vi "level_probe_forhere.vi"(5 "Run VI":bool, 6 "Set # of Turns Open (Man)":dbl, 7 "Target Level (Auto)":dbl format="%.2f", 8 "stop":bool, 9 "Mode":enum32{"AUTOMATIC", "MANUAL"}(radio)=enum."MANUAL", 10 "position":refnum<vi>, 11 "level":refnum<vi>) -> ()   [LabVIEW 2015]
uses:
  <vilib>/Utility/config.llb/Read Key (String).vi
  <vilib>/Utility/config.llb/Read Key (Path).vi
  <vilib>/Utility/file.llb/Read Delimited Spreadsheet (DBL).vi
  <vilib>/Utility/file.llb/Write Delimited Spreadsheet (DBL).vi
  subvi_motor/global_motor.vi
  <vilib>/addons/control/pid/NI_PID_autopid.lvlib
  <vilib>/Utility/config.llb/NI_LVConfig.lvlib
panel:
  out "read buffer":string
  in  "Mode 2":enum32{"Continuous", "Sample and Hold"}(radio)
  in  "Motor Enabled":bool=TRUE
  out "levelbuffer":string
  out "Level":dbl(slide) scale=0.0..100.0
  in  "Save PID gains":bool
  in  "Load PID gains":bool
  in  "Recalibrate":bool
  in  "Current Position":dbl
  out "Motor Connected":bool
  in  "Enable Advanced Controls":bool
  in  "Log Data?":bool
  out "maxsteps":dbl
  out "minsteps":dbl
  in  "Min Open (Auto)":dbl=0.25
  in  "Max Open (Auto)":dbl=0.75
  out "Level":dynamicdata(graph)
  out "Error":dynamicdata(graph)
  in  "PID gains":T1={"proportional gain (Kc)"=10.0, "integral time (Ti, min)"=0.002, "derivative time (Td, min)"=0.2} {"derivative time (Td, min)" format="%.3f"; "integral time (Ti, min)" format="%.3f"; "proportional gain (Kc)" format="%.3f"}
  out "Valve Position":dynamicdata(graph)
  out "# of Turns Open":dbl
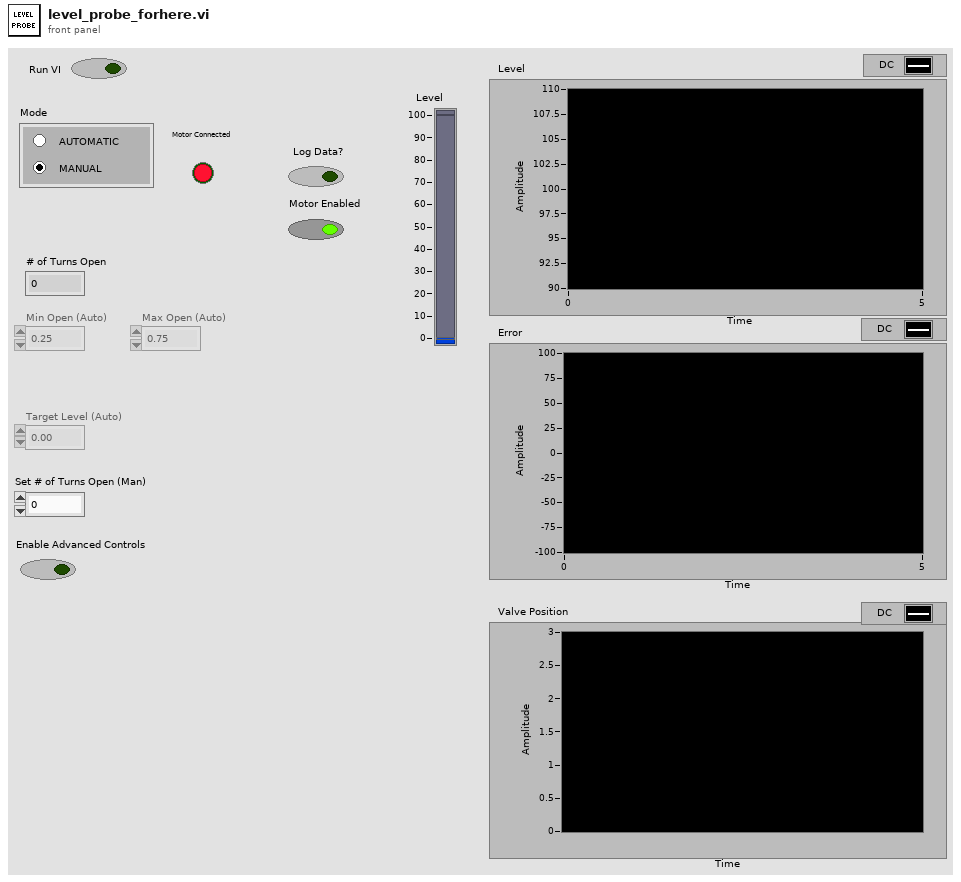
[diagram p1: front panel]
types:
  T1 = cluster{"proportional gain (Kc)":dbl, "integral time (Ti, min)":dbl, "derivative time (Td, min)":dbl}
  T2 = enum16{"open", "replace", "create", "open or create", "replace or create", "replace or create with confirmation"}
  T3 = enum8{"Enabled", "Disabled", "Disabled and Grayed Out"}
  T4 = typedef "NI_LVConfig.lvlib/Config Data RefNum.ctl" = refnum<k1>
  T5 = cluster{"first row[0]":dbl, "first row[1]":dbl, "first row[2]":dbl, "first row[3]":dbl, "first row[4]":dbl, "first row[5]":dbl, "first row[6]":dbl, "first row[7]":dbl, "first row[8]":dbl}
  T6 = cluster{"first row[0]":dbl, "first row[1]":dbl, "first row[2]":dbl}
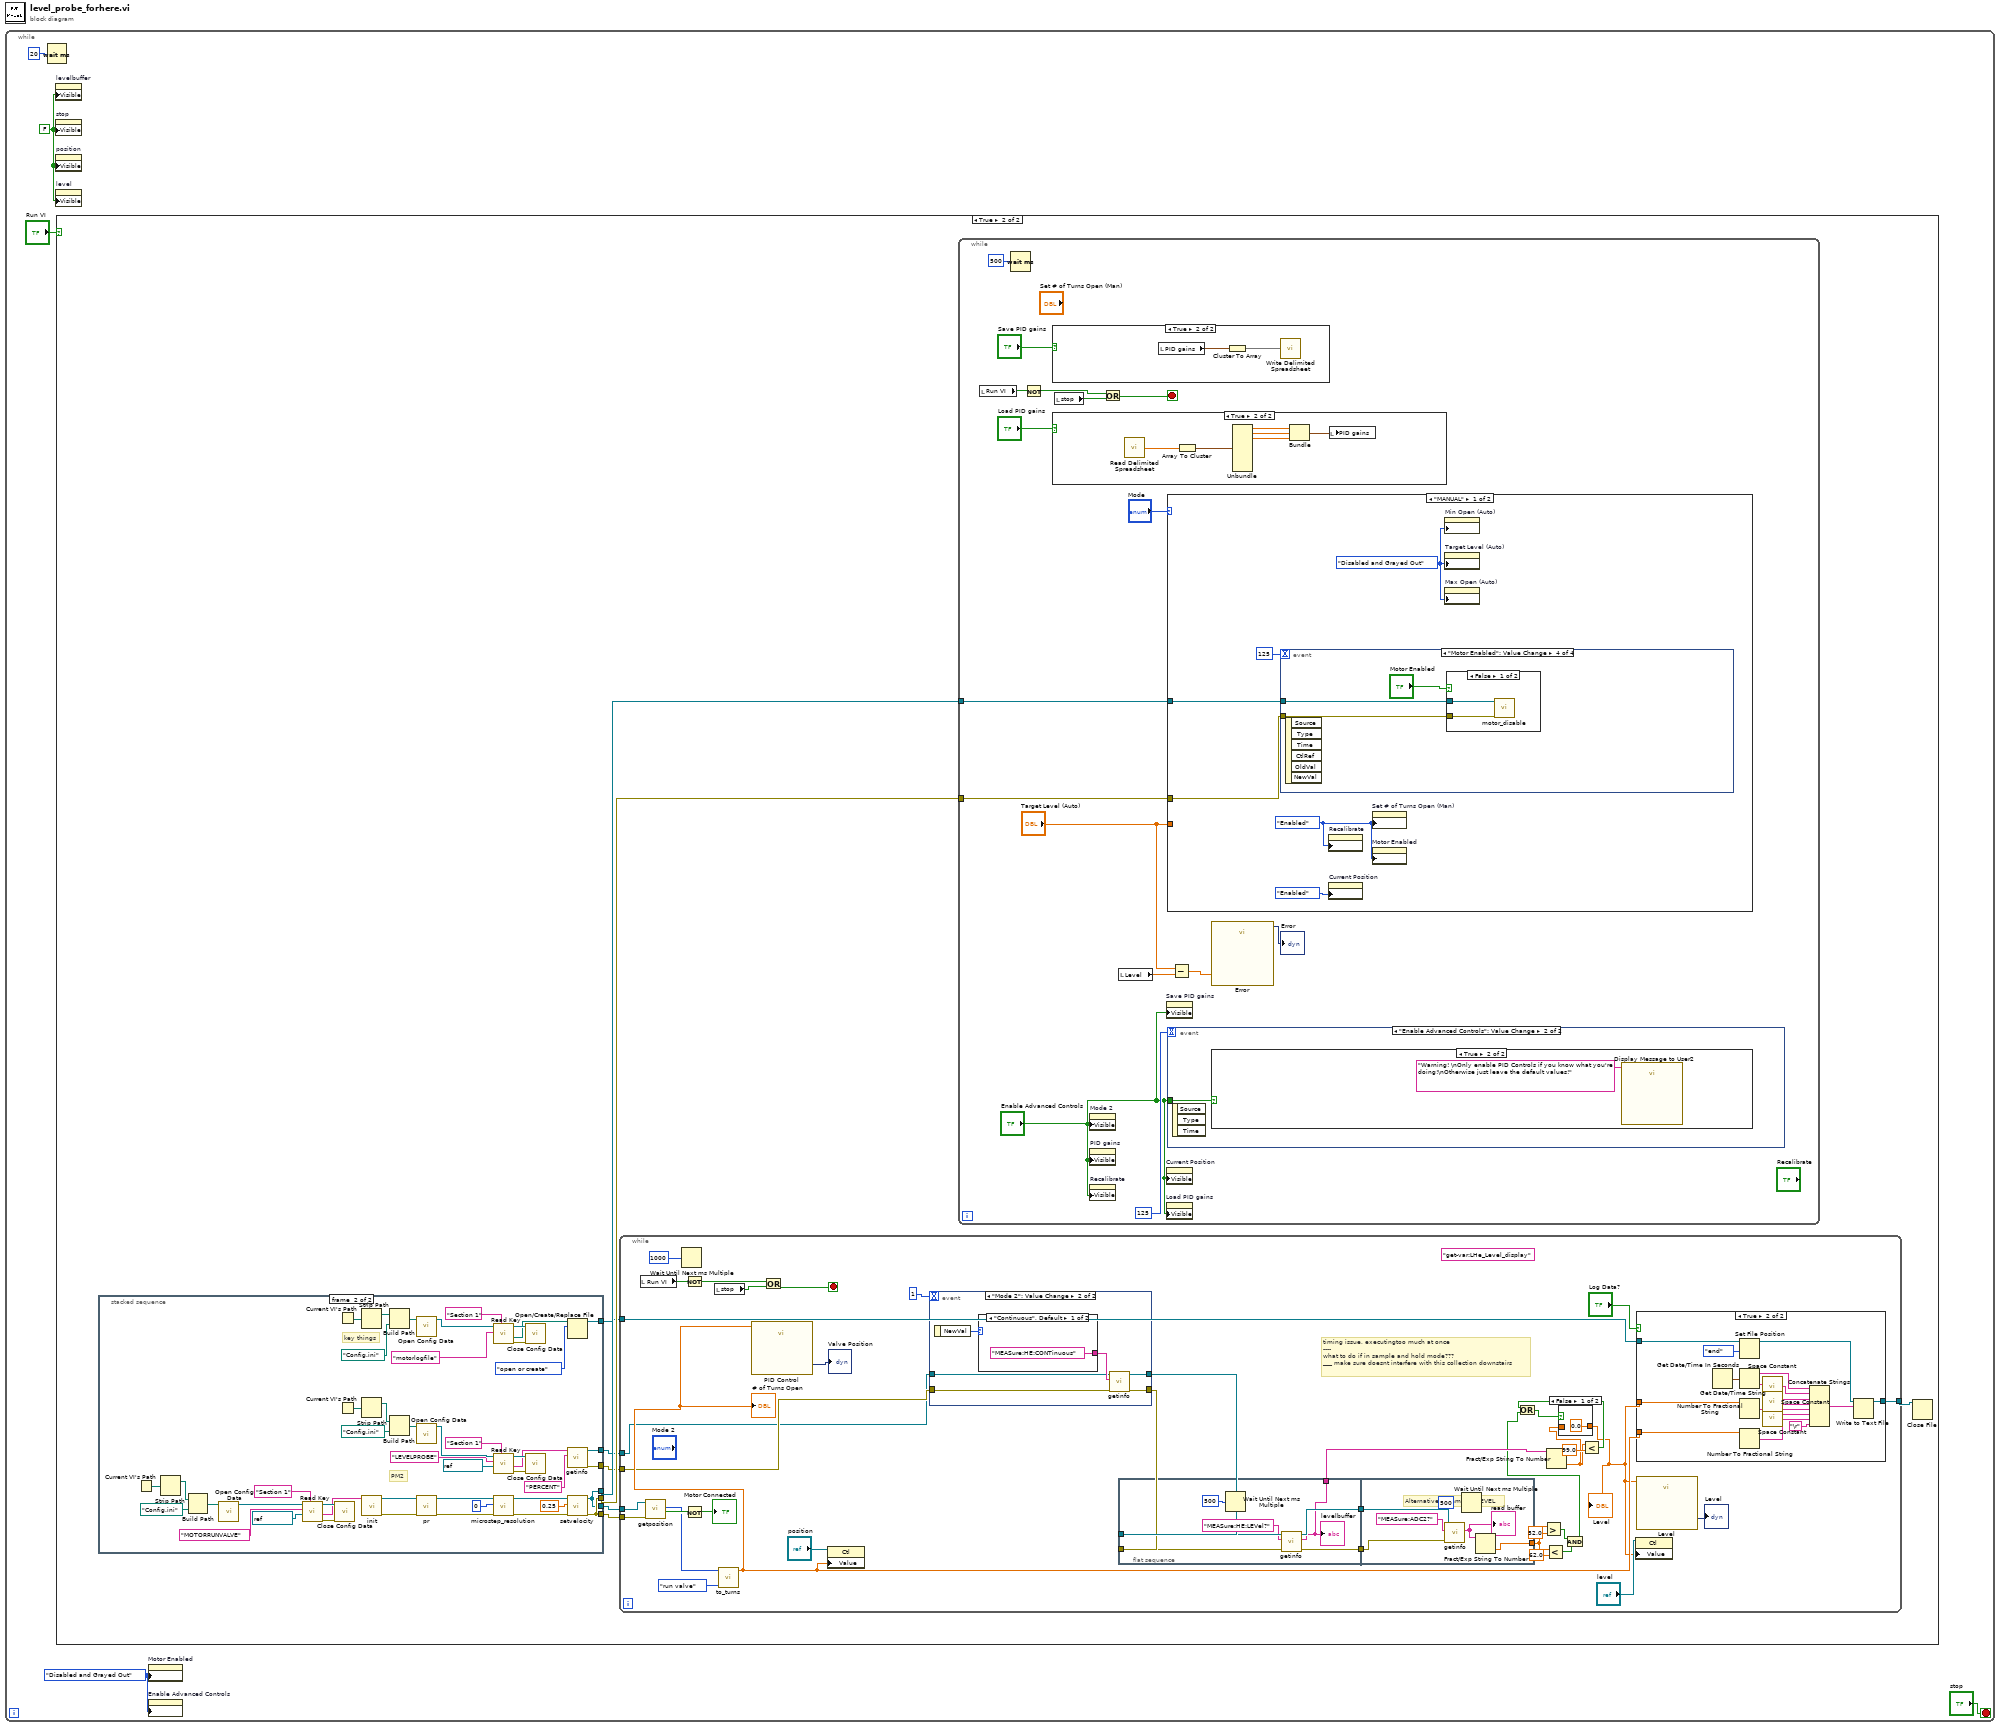
[diagram p0: block diagram]
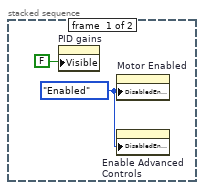
[diagram p3: hidden frame]
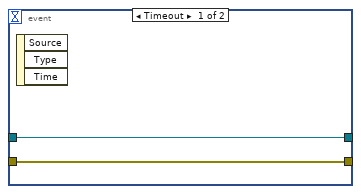
[diagram p5: hidden frame]
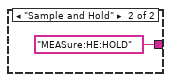
[diagram p6: hidden frame]
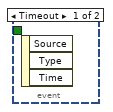
[diagram p8: hidden frame]
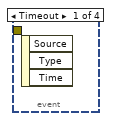
[diagram p12: hidden frame]
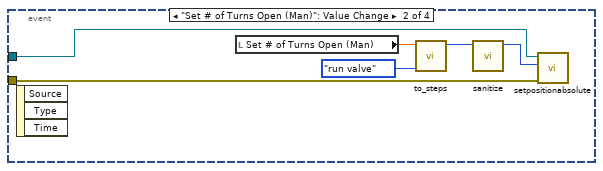
[diagram p13: hidden frame]
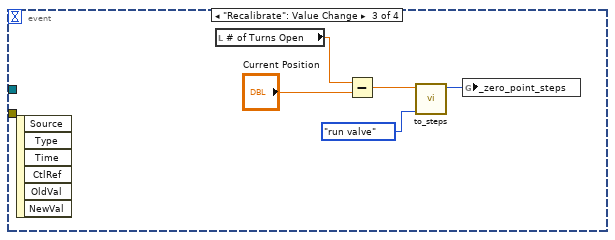
[diagram p14: hidden frame]
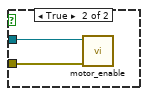
[diagram p15: hidden frame]
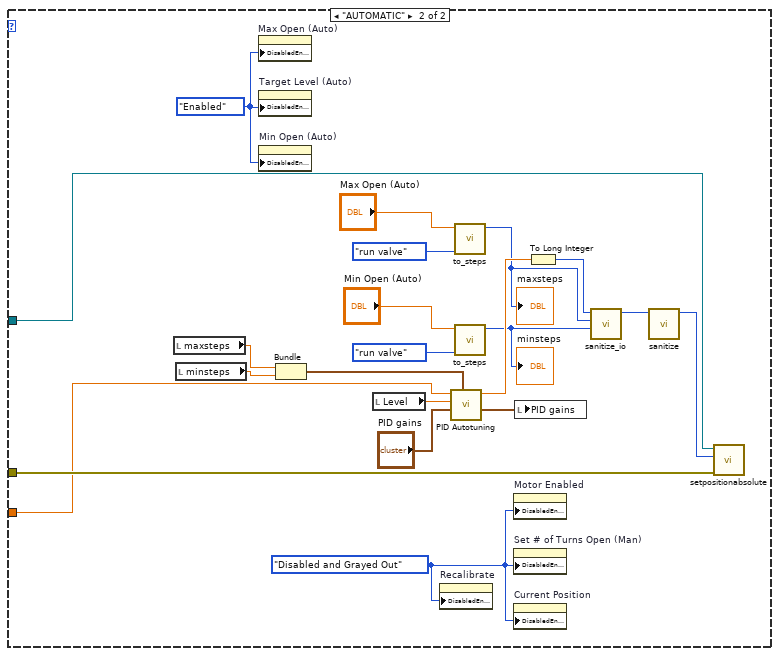
[diagram p16: hidden frame]
diagram:
  n1 = while {
    stop <- "stop" stop-if-true
    w1 = FALSE ("Visible")
    w2 = T3."Disabled and Grayed Out" ("Disabled")
    n2 = Wait (ms)(milliseconds to wait=u32 20) -> ()  [unwired: 1 out]
    n3 = property on="levelbuffer" class="Str"("Visible"=w1) -> ()  [unwired: 2 in, 2 out]
    n4 = property on="stop" class="Bool (strict)"("Visible"=w1) -> ()  [unwired: 2 in, 2 out]
    n5 = property on="position" class="LVObjRef (strict)"("Visible"=w1) -> ()  [unwired: 2 in, 2 out]
    n6 = property on="level" class="LVObjRef (strict)"("Visible"=w1) -> ()  [unwired: 2 in, 2 out]
    n7 = case shown="True" "Run VI" {
      frame False {
      }
      frame True {
        n8 = stacked-sequence {
          tunnel: [_ w61] -> w13
          tunnel: [_ w61] -> w12
          tunnel: [_ w60] -> w11
          tunnel: [_ w60] -> w10
          tunnel: [_ w55] -> w9
          tunnel: [_ w54] -> w8
          tunnel: [_ w53] -> w7
          frame #0 {
            w14 = T3."Enabled" ("Disabled")
            n9 = property on="PID gains" class="Clust (strict)"("Visible"=FALSE) -> ()  [unwired: 2 in, 2 out]
            n10 = property on="Motor Enabled" class="Bool (strict)"("DisabledEnum"=w14) -> ()  [unwired: 2 in, 2 out]
            n11 = property on="Enable Advanced Controls" class="Bool (strict)"("DisabledEnum"=w14) -> ()  [unwired: 2 in, 2 out]
          }
          frame #1 {
            # "PM2"
            # "key things"
            n12 = Current VI's Path() -> (path=w39:path)
            n13 = Strip Path(path=w39) -> (stripped path=w38:path)  [unwired: 1 out]
            n14 = Build Path(base path=w38, name or relative path=path "Config.ini" ("default name")) -> (appended path=w42:path)
            n15 = call <vilib>:"Open Config Data.vi"("configuration file path"=w42) -> ("refnum"=w47:T4)  [unwired: 8 in, 2 out]
            n16 = call-poly <vilib>:"Read Key.vi"("section"="Section 1", "default value"=refnum<visa-resource-name> "COM5" ("VISA resource name"), "key"="MOTORRUNVALVE", "refnum"=w47) -> ("error out"=w41:errorcluster, "value"=w37:string, "refnum out"=w45:T4)  [unwired: 4 in, 1 out]
            n17 = call <vilib>:"Close Config Data.vi"("error in (no error)"=w41, "refnum"=w45) -> ()  [unwired: 8 in, 2 out]
            n18 = Current VI's Path() -> (path=w19:path)
            n19 = Current VI's Path() -> (path=w28:path)
            n20 = Strip Path(path=w19) -> (stripped path=w18:path)  [unwired: 1 out]
            n21 = Strip Path(path=w28) -> (stripped path=w27:path)  [unwired: 1 out]
            n22 = call "init.vi"("VISA resource name"=w37) -> ("error out"=w49:errorcluster, "VISA resource name 2"=w51:refnum<visa-resource-name>)  [unwired: 9 in]
            n23 = Build Path(base path=w18, name or relative path=path "Config.ini" ("default name")) -> (appended path=w21:path)
            n24 = Build Path(base path=w27, name or relative path=path "Config.ini" ("default name")) -> (appended path=w31:path)
            n25 = call <vilib>:"Open Config Data.vi"("configuration file path"=w21) -> ("refnum"=w26:T4)  [unwired: 8 in, 2 out]
            n26 = call <vilib>:"Open Config Data.vi"("configuration file path"=w31) -> ("refnum"=w36:T4)  [unwired: 8 in, 2 out]
            n27 = call "pr.vi"("error in (no error)"=w49, "VISA resource name"=w51) -> ("error out"=w48:errorcluster, "VISA resource name 2"=w50:refnum<visa-resource-name>)  [unwired: 8 in]
            n28 = call-poly <vilib>:"Read Key.vi"("section"="Section 1", "key"="motorlogfile", "refnum"=w26) -> ("error out"=w20:errorcluster, "value"=w17:path, "refnum out"=w24:T4)  [unwired: 5 in, 1 out]
            n29 = call-poly <vilib>:"Read Key.vi"("section"="Section 1", "default value"=refnum<visa-resource-name> "COM8" ("VISA resource name"), "key"="LEVELPROBE", "refnum"=w36) -> ("error out"=w30:errorcluster, "value"=w16:string, "refnum out"=w34:T4)  [unwired: 4 in, 1 out]
            n30 = call "microstep_resolution.vi"("error in (no error)"=w48, "number"=0, "VISA in"=w50) -> ("error out"=w58:errorcluster, "VISA out"=w57:refnum<visa-resource-name>)  [unwired: 7 in]
            n31 = call <vilib>:"Close Config Data.vi"("error in (no error)"=w20, "refnum"=w24) -> ()  [unwired: 8 in, 2 out]
            n32 = call <vilib>:"Close Config Data.vi"("error in (no error)"=w30, "refnum"=w34) -> ()  [unwired: 8 in, 2 out]
            n33 = Open/Create/Replace File(file path (use dialog)=w17, operation (0:open)=T2."open or create") -> (refnum out=w53:refnum<file>)  [unwired: 4 in, 2 out]
            n34 = call "getinfo.vi"("string"="PERCENT", "VISA resource name"=w16) -> ("error out"=w54:errorcluster, "VISA resource name 2"=w55:refnum<visa-resource-name>)  [unwired: 7 in, 1 out]
            n35 = call "setvelocity.vi"("error in (no error)"=w58, "Velocity"=0.25, "VISA in"=w57) -> ("error out"=w61:errorcluster, "VISA out"=w60:refnum<visa-resource-name>)  [unwired: 7 in]
          }
        }
        n36 = while {
          tunnel: w12 -> [w100]
          tunnel: w10 -> [w99]
          tunnel: w9 -> [w80]
          tunnel: w8 -> [w81]
          tunnel: w7 -> [w85]
          tunnel: [w84] -> w6
          stop <- w87 stop-if-true
          (unwired) "get-var:LHe_Level_display" ("string")
          # "timing issue, executingtoo much at once\n----\nwhat to do if in sample and hold mode???\n___ make sure doesnt interfere with this collection downstairs"
          # "Alternative Command: LEVEL"
          n37 = local read "Run VI"() -> (w92:bool)
          n38 = call "getposition.vi"("error in (no error)"=w100, "VISA resource name"=w99) -> ("Is Null?"=w95:bool, "Position"=w93:i32)  [unwired: 6 in, 2 out]
          n39 = Wait Until Next ms Multiple(millisecond multiple=u32 1000 ("milliseconds to wait")) -> ()  [unwired: 1 out]
          n40 = Not(x=w92) -> (.not. x?=w88:bool)
          n41 = Not(x=w95) -> (.not. x?=→"Motor Connected":bool)
          n42 = local read "stop"() -> (w86:bool)
          n43 = call "to_turns.vi"("Radio Buttons"=enum32{"run valve", "bypass valve"}."run valve", "Steps"=w93) -> ("Turns"=w89:dbl)  [unwired: 9 in]
          "# of Turns Open" <- w89
          n44 = call "PID Control"("Offset"=w89) -> ("DC"=→"Valve Position":dynamicdata)  [unwired: 13 in, 1 out]
          n45 = Or(x=w88, y=w86) -> (x .or. y?=w87:bool)
          n46 = property class="Ctl"(reference="position", "Value"=w89) -> ()  [unwired: 1 in, 2 out]
          n47 = event shown="[1] \"Mode 2\": Value Change" {
            selector: _ -> [_ _]
            dyn-events: _ -> [_ _]
            timeout: 1 -> [_ _]
            tunnel: w81 -> [w116 w120]
            tunnel: w80 -> [w117 w121]
            tunnel: [w117 w119] -> w79
            tunnel: [w116 w118] -> w78
            event Timeout {
              n48 = event-data() -> ()  [unwired: 1 in, 3 out]
            }
            event "Mode 2": Value Change {
              n49 = event-data() -> ("NewVal"=w123:enum32{"Continuous", "Sample and Hold"})  [unwired: 1 in]
              n50 = case shown="\"Continuous\", Default" w123 {
                tunnel: ["MEASure:HE:CONTinuous" ("string") "MEASure:HE:HOLD"] -> w122
                frame "Continuous", Default {
                }
                frame "Sample and Hold" {
                }
              }
              n51 = call "getinfo.vi"("error in (no error)"=w120, "string"=w122, "VISA resource name"=w121) -> ("error out"=w118:errorcluster, "VISA resource name 2"=w119:refnum<visa-resource-name>)  [unwired: 6 in, 1 out]
            }
          }
          n52 = flat-sequence {
            tunnel: w79 -> [w109]
            tunnel: w78 -> [w107]
            tunnel: [w105] -> w76
            tunnel: [w104] -> w75
            tunnel: [w103] -> w74
            tunnel: w76 -> [w114]
            tunnel: w75 -> [w113]
            tunnel: [w110] -> w72
            frame #0 {
              n53 = Wait Until Next ms Multiple(millisecond multiple=u32 500) -> ()  [unwired: 1 out]
              n54 = call "getinfo.vi"("error in (no error)"=w107, "string"="MEASure:HE:LEVel?", "VISA resource name"=w109) -> ("error out"=w104:errorcluster, "read buffer"=w103:string, "VISA resource name 2"=w105:refnum<visa-resource-name>)  [unwired: 6 in]
              "levelbuffer" <- w103
            }
            frame #1 {
              n55 = call "getinfo.vi"("error in (no error)"=w113, "string"="MEASure:ADC2?", "VISA resource name"=w114) -> ("read buffer"=w111:string)  [unwired: 6 in, 2 out]
              "read buffer" <- w111
              n56 = Wait Until Next ms Multiple(millisecond multiple=u32 500) -> ()  [unwired: 1 out]
              n57 = Fract/Exp String To Number(string=w111) -> (number=w110:dbl)  [unwired: 3 in, 1 out]
            }
          }
          n58 = Greater?(x=w72, y=52.0) -> (0:w70:bool)
          n59 = Less?(x=w72, y=62.0) -> (x < y?=w69:bool)
          n60 = Fract/Exp String To Number(string=w74) -> (number=w64:dbl)  [unwired: 3 in, 1 out]
          n61 = And(x=w70, y=w69) -> (x .and. y?=w66:bool)
          n62 = Less?(x=w64, y=99.0) -> (x < y?=w67:bool)
          n63 = Or(x=w67, y=w66) -> (x .or. y?=w63:bool)
          n64 = case shown="False" w63 {
            tunnel: [0.0 w102] -> w65
            tunnel: w64 -> [_ w102]
            frame False {
            }
            frame True {
            }
          }
          "Level" <- w65
          n65 = property class="Ctl"(reference="level", "Value"=w65) -> ()  [unwired: 1 in, 2 out]
          n66 = case shown="True" "Log Data?" {
            tunnel: w89 -> [_ w142]
            tunnel: w65 -> [_ w137]
            tunnel: w85 -> [w126 w132]
            tunnel: [w126 w131] -> w84
            frame False {
            }
            frame True {
              n67 = Get Date/Time In Seconds() -> (seconds since 1Jan1904=w130:timestamp)
              n68 = Set File Position(refnum=w132, from (0:start)=enum16{"start", "end", "current"}."end") -> (refnum out=w138:refnum<file>)  [unwired: 2 in, 1 out]
              n69 = Get Date/Time String(seconds (now)=w130) -> (date string=w128:string, time string=w129:string)  [unwired: 2 in]
              n70 = Number To Fractional String(number=w137) -> (F-format string=w136:string)  [unwired: 3 in]
              n71 = Number To Fractional String(number=w142) -> (F-format string=w134:string)  [unwired: 3 in]
              n72 = call <vilib>:"Space Constant.vi"() -> ("String"=w127:string)
              n73 = call <vilib>:"Space Constant.vi"() -> ("String"=w140:string)
              n74 = call <vilib>:"Space Constant.vi"() -> ("String"=w135:string)
              n75 = Concatenate Strings(w128, w127, w129, w140, w136, w135, w134, "\r") -> (w141:string)
              n76 = Write to Text File(file (use dialog)=w138, text=w141) -> (refnum out=w131:refnum<file>)  [unwired: 2 in, 2 out]
            }
          }
          n77 = call "Level"("Offset"=w65) -> ("DC"=→"Level":dynamicdata)  [unwired: 13 in, 1 out]
        }
        n78 = while {
          tunnel: w13 -> [w157]
          tunnel: w11 -> [w156]
          stop <- w145 stop-if-true
          n79 = local read "Run VI"() -> (w148:bool)
          n80 = Wait (ms)(milliseconds to wait=u32 500) -> ()  [unwired: 1 out]
          n81 = Not(x=w148) -> (.not. x?=w146:bool)
          n82 = case shown="True" "Save PID gains" {
            frame False {
            }
            frame True {
              n83 = local read "PID gains"() -> (w162:T1)
              n84 = Cluster To Array(cluster=w162) -> (array=w161:dbl[])
              n85 = call-poly <vilib>:"Write Delimited Spreadsheet.vi"("1D data"=w161) -> ()  [unwired: 13 in, 2 out]
            }
          }
          n86 = case shown="True" "Load PID gains" {
            frame False {
            }
            frame True {
              n87 = call-poly <vilib>:"Read Delimited Spreadsheet.vi"() -> ("first row"=w168:dbl[])  [unwired: 10 in, 5 out]
              n88 = Array To Cluster(array=w168) -> (cluster=w167:T5)
              n89 = Unbundle(w167) -> ("first row[0]"=w166:dbl, "first row[1]"=w165:dbl, "first row[2]"=w164:dbl)  [unwired: 6 out]
              n90 = Bundle("first row[0]"=w166, "first row[1]"=w165, "first row[2]"=w164) -> (w163:T6)  [unwired: 1 in]
              n91 = local write "PID gains"(w163) -> ()
            }
          }
          n92 = local read "stop"() -> (w144:bool)
          n93 = property on="Mode 2" class="RadioBtnsControl (strict)"("Visible"="Enable Advanced Controls") -> ()  [unwired: 2 in, 2 out]
          n94 = property on="PID gains" class="Clust (strict)"("Visible"="Enable Advanced Controls") -> ()  [unwired: 2 in, 2 out]
          n95 = property on="Recalibrate" class="Bool"("Visible"="Enable Advanced Controls") -> ()  [unwired: 2 in, 2 out]
          n96 = Or(x=w146, y=w144) -> (x .or. y?=w145:bool)
          n97 = local read "Level"() -> (w147:dbl)
          n98 = property on="Save PID gains" class="Bool"("Visible"="Enable Advanced Controls") -> ()  [unwired: 2 in, 2 out]
          n99 = property on="Current Position" class="DigNum (strict)"("Visible"="Enable Advanced Controls") -> ()  [unwired: 2 in, 2 out]
          n100 = property on="Load PID gains" class="Bool"("Visible"="Enable Advanced Controls") -> ()  [unwired: 2 in, 2 out]
          n101 = case shown="\"MANUAL\"" "Mode" {
            tunnel: w156 -> [w174 w210]
            tunnel: w157 -> [w173 w211]
            tunnel: "Target Level (Auto)" -> [_ w209]
            frame "MANUAL" {
              w170 = T3."Enabled" ("Disabled")
              w169 = T3."Disabled and Grayed Out" ("Disabled")
              n102 = event shown="[3] \"Motor Enabled\": Value Change" {
                selector: _ -> [_ _ _ _]
                dyn-events: _ -> [_ _ _ _]
                timeout: 125 -> [_ _ _ _]
                tunnel: w174 -> [_ w179 _ w188]
                tunnel: w173 -> [_ w178 _ w187]
                event Timeout {
                  n103 = event-data() -> ()  [unwired: 1 in, 3 out]
                }
                event "Set # of Turns Open (Man)": Value Change {
                  n104 = event-data() -> ()  [unwired: 1 in, 3 out]
                  n105 = local read "Set # of Turns Open (Man)"() -> (w177:dbl)
                  n106 = call "to_steps.vi"("Radio Buttons"=enum32{"run valve", "bypass valve"}."run valve", "Turns"=w177) -> ("Steps"=w176:i32)  [unwired: 9 in]
                  n107 = call "sanitize.vi"("Input"=w176) -> ("Sanitized Input"=w180:i32)  [unwired: 10 in]
                  n108 = call "setpositionabsolute.vi"("error in (no error)"=w178, "Position Aboslute"=w180, "VISA in"=w179) -> ()  [unwired: 7 in, 2 out]
                }
                event "Recalibrate": Value Change {
                  n109 = event-data() -> ()  [unwired: 1 in, 6 out]
                  n110 = local read "# of Turns Open"() -> (w183:dbl)
                  n111 = Subtract(x=w183, y="Current Position") -> (x-y=w184:dbl)
                  n112 = call "to_steps.vi"("Radio Buttons"=enum32{"run valve", "bypass valve"}."run valve", "Turns"=w184) -> ("Steps"=w185:i32)  [unwired: 9 in]
                  n113 = global write "global_motor.vi" "_zero_point_steps"(w185) -> ()
                }
                event "Motor Enabled": Value Change {
                  n114 = event-data() -> ()  [unwired: 1 in, 6 out]
                  n115 = case shown="False" "Motor Enabled" {
                    tunnel: w188 -> [w189 w192]
                    tunnel: w187 -> [w190 w191]
                    frame False {
                      n116 = call "motor_disable.vi"("error in (no error)"=w190, "VISA resource name"=w189) -> ()  [unwired: 8 in, 2 out]
                    }
                    frame True {
                      n117 = call "motor_enable.vi"("error in (no error)"=w191, "VISA resource name"=w192) -> ()  [unwired: 8 in, 2 out]
                    }
                  }
                }
              }
              n118 = property on="Recalibrate" class="Bool"("DisabledEnum"=w170) -> ()  [unwired: 2 in, 2 out]
              n119 = property on="Current Position" class="DigNum (strict)"("DisabledEnum"=T3."Enabled" ("Disabled")) -> ()  [unwired: 2 in, 2 out]
              n120 = property on="Set # of Turns Open (Man)" class="DigNum (strict)"("DisabledEnum"=w170) -> ()  [unwired: 2 in, 2 out]
              n121 = property on="Motor Enabled" class="Bool (strict)"("DisabledEnum"=w170) -> ()  [unwired: 2 in, 2 out]
              n122 = property on="Min Open (Auto)" class="DigNum (strict)"("DisabledEnum"=w169) -> ()  [unwired: 2 in, 2 out]
              n123 = property on="Target Level (Auto)" class="DigNum (strict)"("DisabledEnum"=w169) -> ()  [unwired: 2 in, 2 out]
              n124 = property on="Max Open (Auto)" class="DigNum (strict)"("DisabledEnum"=w169) -> ()  [unwired: 2 in, 2 out]
            }
            frame "AUTOMATIC" {
              w196 = T3."Disabled and Grayed Out" ("Disabled")
              w195 = T3."Enabled" ("Disabled")
              n125 = local read "maxsteps"() -> (w208:dbl)
              n126 = local read "minsteps"() -> (w207:dbl)
              n127 = property on="Max Open (Auto)" class="DigNum (strict)"("DisabledEnum"=w195) -> ()  [unwired: 2 in, 2 out]
              n128 = property on="Target Level (Auto)" class="DigNum (strict)"("DisabledEnum"=w195) -> ()  [unwired: 2 in, 2 out]
              n129 = property on="Min Open (Auto)" class="DigNum (strict)"("DisabledEnum"=w195) -> ()  [unwired: 2 in, 2 out]
              n130 = Bundle("maxsteps"=w208, "minsteps"=w207) -> (w201:cluster{"maxsteps":dbl, "minsteps":dbl})  [unwired: 1 in]
              n131 = local read "Level"() -> (w197:dbl)
              n132 = property on="Recalibrate" class="Bool"("DisabledEnum"=w196) -> ()  [unwired: 2 in, 2 out]
              n133 = call <vilib>:"PID Autotuning.vi"("output range"=w201, "PID gains"="PID gains", "process variable"=w197, "setpoint"=w209) -> ("PID gains out"=w200:T1, "output"=w212:dbl)  [unwired: 4 in, 2 out]
              n134 = call "to_steps.vi"("Radio Buttons"=enum32{"run valve", "bypass valve"}."run valve", "Turns"="Max Open (Auto)") -> ("Steps"=w203:i32)  [unwired: 9 in]
              "maxsteps" <- w203
              n135 = call "to_steps.vi"("Radio Buttons"=enum32{"run valve", "bypass valve"}."run valve", "Turns"="Min Open (Auto)") -> ("Steps"=w202:i32)  [unwired: 9 in]
              "minsteps" <- w202
              n136 = property on="Motor Enabled" class="Bool (strict)"("DisabledEnum"=w196) -> ()  [unwired: 2 in, 2 out]
              n137 = property on="Set # of Turns Open (Man)" class="DigNum (strict)"("DisabledEnum"=w196) -> ()  [unwired: 2 in, 2 out]
              n138 = property on="Current Position" class="DigNum (strict)"("DisabledEnum"=w196) -> ()  [unwired: 2 in, 2 out]
              n139 = local write "PID gains"(w200) -> ()
              n140 = To Long Integer(number=w212) -> (32bit integer=w206:i32)
              n141 = call "sanitize_io.vi"("min"=w202, "max"=w203, "Input"=w206) -> ("Sanitized Input"=w198:i32)  [unwired: 8 in]
              n142 = call "sanitize.vi"("Input"=w198) -> ("Sanitized Input"=w199:i32)  [unwired: 10 in]
              n143 = call "setpositionabsolute.vi"("error in (no error)"=w211, "Position Aboslute"=w199, "VISA in"=w210) -> ()  [unwired: 7 in, 2 out]
            }
          }
          n144 = event shown="[1] \"Enable Advanced Controls\": Value Change" {
            selector: _ -> [_ _]
            dyn-events: _ -> [_ _]
            timeout: 125 -> [_ _]
            tunnel: "Enable Advanced Controls" -> [_ w159]
            event Timeout {
              n145 = event-data() -> ()  [unwired: 1 in, 3 out]
            }
            event "Enable Advanced Controls": Value Change {
              n146 = event-data() -> ()  [unwired: 1 in, 3 out]
              n147 = case shown="True" w159 {
                frame False {
                }
                frame True {
                  n148 = call "Display Message to User2"("Message"="Warning! \nOnly enable PID Controls if you know what you're doing!\nOtherwise just leave the default values!") -> ()  [unwired: 9 in, 2 out]
                }
              }
            }
          }
          n149 = Subtract(x="Target Level (Auto)", y=w147) -> (x-y=w153:dbl)
          n150 = call "Error"("Offset"=w153) -> ("DC"=→"Error":dynamicdata)  [unwired: 13 in, 1 out]
        }
        n151 = Close File(refnum=w6) -> ()  [unwired: 1 in, 2 out]
      }
    }
    n152 = property on="Motor Enabled" class="Bool (strict)"("DisabledEnum"=w2) -> ()  [unwired: 2 in, 2 out]
    n153 = property on="Enable Advanced Controls" class="Bool (strict)"("DisabledEnum"=w2) -> ()  [unwired: 2 in, 2 out]
  }
